vi "Get one MathCAD design.vi"(8 "error in (no error)":errorcluster) -> (0 "error out":errorcluster, 1 "DesignRequest":T2, 2 "Find-Replace":cluster{"Find":string, "Replace":string}[](array[cluster]), 3 "Mathcad Output":T1, 4 "Number of Pending Requests":i32)   [LabVIEW 2011, in "Design Server.lvlib"]
uses:
  Design Server.lvlib
  Design Request.ctl
  Variable cluster.ctl
panel:
  in  "Clust Refnum 2":refnum<vi>
  in  "Clust Refnum":refnum<vi>
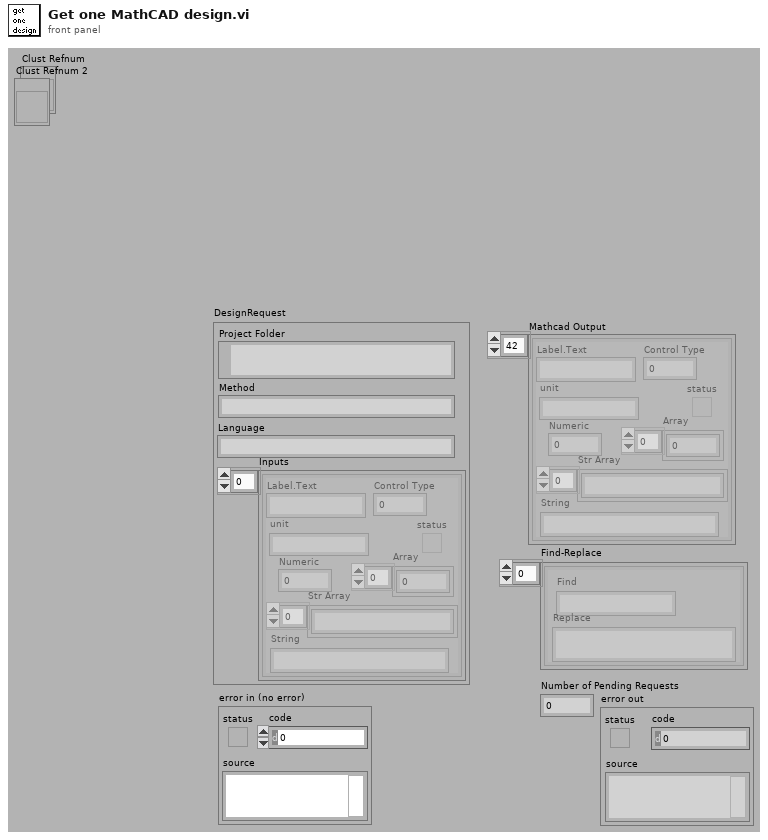
[diagram p1: front panel]
types:
  T1 = typedef "Design Server.lvlib/Variable cluster.ctl" = cluster{"Label.Text":string, "Control Type":u32, "Numeric":dbl, "Array":dbl[], "status":bool, "Str Array":string[], "String":string, "unit":string}[]
  T2 = typedef "Design Server.lvlib/Design Request.ctl" = cluster{"Project Folder":path, "Method":string, "Inputs":T1, "Language":string}
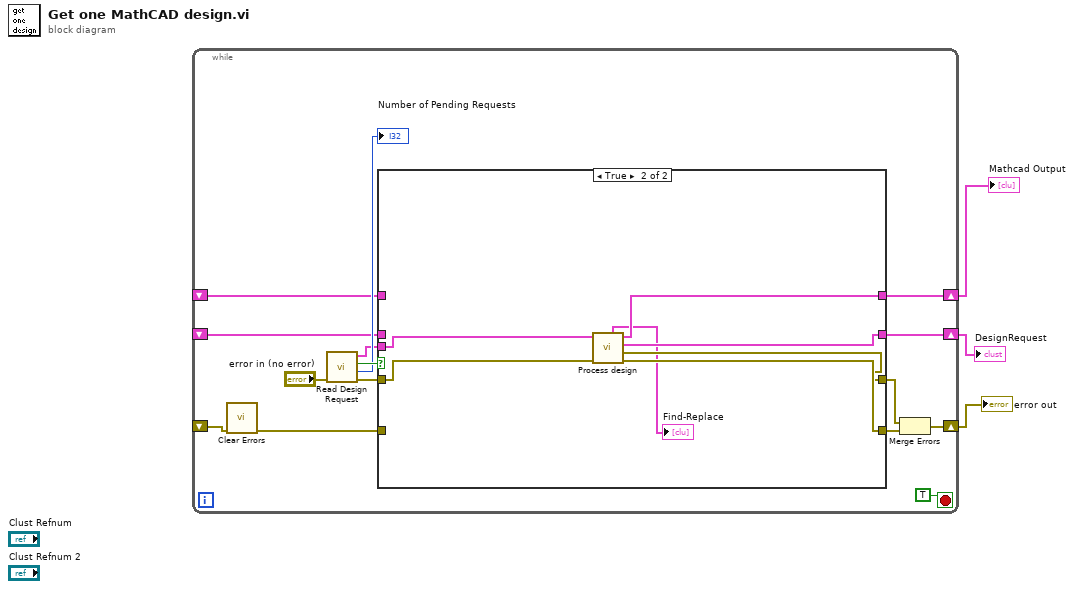
[diagram p0: block diagram]
diagram:
  n1 = while {
    shift-right: [w12] -> w3
    shift-left: _ -> [w11]
    shift-right: [w10] -> w2
    shift-left: _ -> [w9]
    shift-right: [w6] -> w1
    shift-left: _ -> [w5]
    stop <- TRUE stop-if-true
    n2 = call <vilib>:"Clear Errors.vi"("error in (no error)"=w5) -> ("error out"=w4:errorcluster)  [unwired: 6 in]
    n3 = call "Read Design Request.vi"("error in"="error in (no error)") -> ("error out"=w16:errorcluster, "Number of Pending Requests"=→"Number of Pending Requests":i32, "Request Pending"=w17:bool, "DesignRequest"=w14:T2)  [unwired: 7 in]
    n4 = case shown="True" w17 {
      tunnel: w16 -> [w22 w29]
      tunnel: w14 -> [_ w28]
      tunnel: [w22 w24] -> w8
      tunnel: [w21 w27] -> w12
      tunnel: w11 -> [w21 _]
      tunnel: [w20 w26] -> w10
      tunnel: w9 -> [w20 _]
      tunnel: [w19 w25] -> w7
      tunnel: w4 -> [w19 _]
      frame False {
      }
      frame True {
        n5 = call "Process design.vi"("error in (no error)"=w29, "DesignRequest"=w28) -> ("design error"=w25:errorcluster, "output error"=w24:errorcluster, "DesignRequest out"=w26:T2, "Mathcad Output"=w27:T1, "Find-Replace"=→"Find-Replace":cluster{"Find":string, "Replace":string}[])  [unwired: 5 in]
      }
    }
    n6 = Merge Errors(w8, w7) -> (w6:errorcluster)
  }
  "Mathcad Output" <- w3
  "DesignRequest" <- w2
  "error out" <- w1
